vi "XIPIN_AXI4-Stream_to_Video_Out_4_0.vi"   [LabVIEW 2017]
doc: "Video bridge converting AXI4-Stream to native video.\n------------------------------------\n<b>Need License</b> : No\n<b>Interface</b> : AXI4-Stream"
uses:
  <vilib>/rvi/XilinxIP/XIPIN_XNode/niFpgaXIPIN.xnode
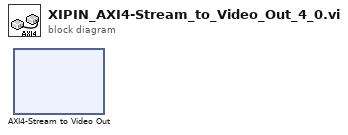
[diagram p0: block diagram]
diagram:
  n1 = xnode ("AXI4-Stream to Video Out")() -> ()
